vi "Initialize.vi"() -> ()   [LabVIEW 2012, in "GoToWaypoint.lvclass"]
uses:
  GoToWaypoint.lvclass
  Sailbot2012_2013/Software/2-Think/2 Typedefs/UTM Location.ctl
panel:
  out "GoToWaypoint Object 2":refnum<class "GoToWaypoint.lvclass">
  in  "Constant Cluster":T2 {"Drive Location"."North" format="%#_10f"; "Drive Location"."East" format="%#_8f"}
  out "Error Out":errorcluster
  in  "Error In":errorcluster
  in  "Tolerance (m)":dbl
  in  "Drive Location":T1 {"North" format="%#_10f"; "East" format="%#_8f"}
  in  "GoToWaypoint Object":refnum<class "GoToWaypoint.lvclass">
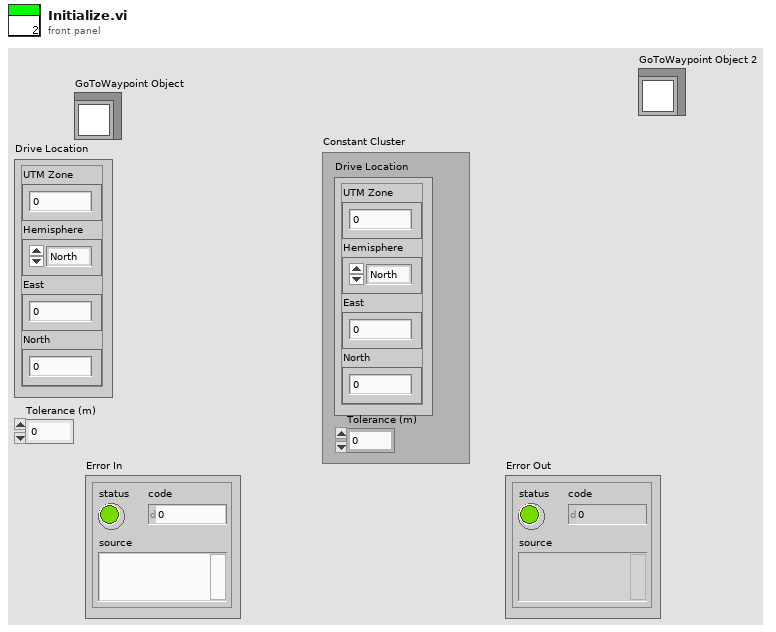
[diagram p1: front panel]
types:
  T1 = typedef "UTM Location.ctl" = cluster{"UTM Zone":dbl, "Hemisphere":enum16{"North", "South"}, "East":dbl, "North":dbl}
  T2 = cluster{"Drive Location":T1, "Tolerance (m)":dbl}
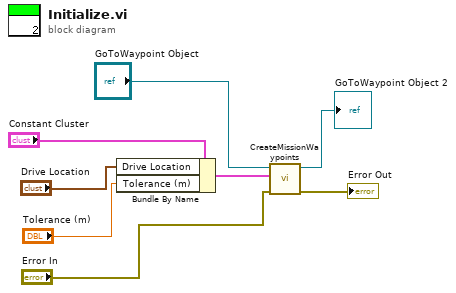
[diagram p0: block diagram]
diagram:
  n1 = Bundle By Name(cluster="Constant Cluster", "Drive Location"="Drive Location", "Tolerance (m)"="Tolerance (m)") -> (w3:T2)
  n2 = call "CreateMissionWaypoints.vi"("error in (no error)"="Error In", "WayPointCluster"=w3, "GoToWaypoint In"="GoToWaypoint Object") -> ("error out"=→"Error Out":errorcluster, "GoToWaypoint Out"=→"GoToWaypoint Object 2":refnum<class "GoToWaypoint.lvclass">)  [unwired: 4 in]
